vi "PhotonVision_ReadData.vi"() -> ()   [LabVIEW 2019]
uses:
  <vilib>/Rock Robotics/WPI/ThirdParty/PhotonVisionLib/TypeDef/PhotonPipelineResultType.ctl
  <vilib>/Rock Robotics/WPI/ThirdParty/PhotonVisionLib/TypeDef/PhotonTrackedTargetType.ctl
  <vilib>/Rock Robotics/WPI/ThirdParty/PhotonVisionLib/TypeDef/TargetCornerType.ctl
  <vilib>/Rock Robotics/WPI/ThirdParty/JAS_Junk/TrajLib/TypeDef/TRANSFORM3D.ctl
  <vilib>/Rock Robotics/WPI/ThirdParty/JAS_Junk/TrajLib/TypeDef/TRANSLATION3D.ctl
  <vilib>/Rock Robotics/WPI/ThirdParty/JAS_Junk/TrajLib/TypeDef/ROTATION3D.ctl
  <vilib>/Rock Robotics/WPI/ThirdParty/JAS_Junk/TrajLib/TypeDef/QUATERNION.ctl
  <vilib>/Rock Robotics/Network Tables/NT Write Boolean.vi
  <vilib>/Rock Robotics/Network Tables/NT Write Number.vi
  <vilib>/Rock Robotics/WPI/ThirdParty/PhotonVisionLib/PhotonVisionLib.lvlib
  <vilib>/Rock Robotics/WPI/ThirdParty/JAS_Junk/TrajLib/Trajectory_Library.lvlib
panel:
  out "IsConnected":bool
  out "Found Targets":bool
  in  "CameraName":string="Microsoft LifeCam HD-3000"
  out "CtrlLibDistToBestTarg\nMeters":dbl
  out "Loop Count":i32
  out "SpecificPhotonTrackedTarget":T1={"Yaw"=0.0, "Pitch"=0.0, "Area"=0.0, "Skew"=0.0, "MinAreaRectCorners"=[], "BestCameraToTarget"={"TRANSLATION3D"={"X"=0.0, "Y"=0.0, "Z"=0.0}, "ROTATION3D"={"Q_quaternion"={"R"=1.0, "V"=[0.0, 0.0, 0.0]}}, "XF"=FALSE}, "FiiducialId"=0, "AltCameraToTarget"={"TRANSLATION3D"={"X"=0.0, "Y"=0.0, "Z"=0.0}, "ROTATION3D"={"Q_quaternion"={"R"=0.0, "V"=[0.0, 0.0, 0.0]}}, "XF"=FALSE}, "PoseAmbiguity"=0.0, "DetectedCorners"=[]} {"AltCameraToTarget"."TRANSLATION3D"."Z" format="%14.3f"; "AltCameraToTarget"."TRANSLATION3D"."Y" format="%14.3f"; "AltCameraToTarget"."TRANSLATION3D"."X" format="%14.3f"; "BestCameraToTarget"."TRANSLATION3D"."Z" format="%14.3f"; "BestCameraToTarget"."TRANSLATION3D"."Y" format="%14.3f"; "BestCameraToTarget"."TRANSLATION3D"."X" format="%14.3f"}
  out "PipelineResult":T7 {"Targets"."AltCameraToTarget"."TRANSLATION3D"."Z" format="%14.3f"; "Targets"."AltCameraToTarget"."TRANSLATION3D"."Y" format="%14.3f"; "Targets"."AltCameraToTarget"."TRANSLATION3D"."X" format="%14.3f"; "Targets"."BestCameraToTarget"."TRANSLATION3D"."Z" format="%14.3f"; "Targets"."BestCameraToTarget"."TRANSLATION3D"."Y" format="%14.3f"; "Targets"."BestCameraToTarget"."TRANSLATION3D"."X" format="%14.3f"}
  out "SpecificTargetFound":bool
  out "TagTarget Index":i32
  in  "Fiiducial ID\n(April Tag Number)":i32
  out "BestTargetFound":bool
  out "BestYaw":dbl
  out "DistanceToBestTarget \nMeters":dbl
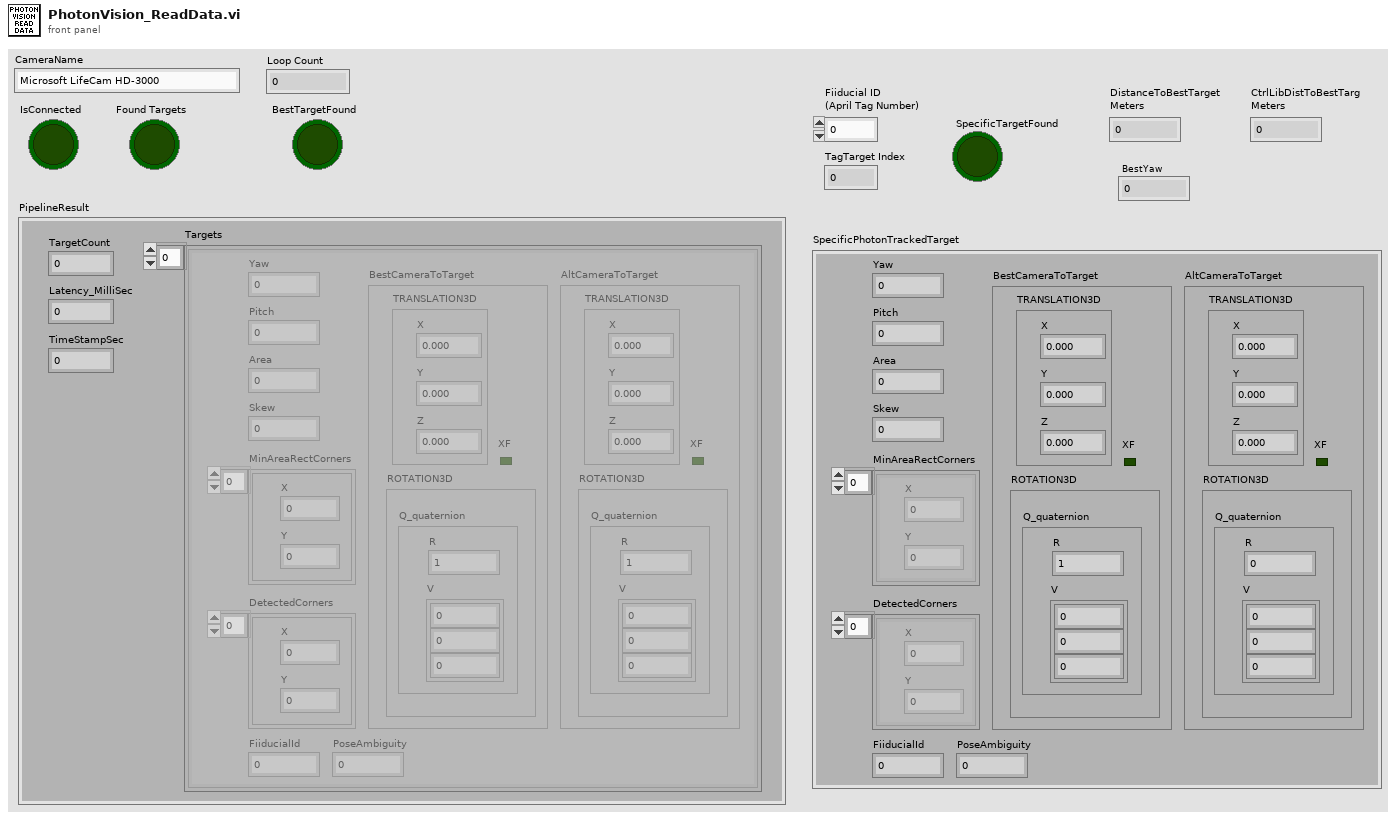
[diagram p1: front panel]
types:
  T1 = typedef "PhotonVisionLib.lvlib/PhotonTrackedTargetType.ctl" = cluster{"Yaw":dbl, "Pitch":dbl, "Area":dbl, "Skew":dbl, "MinAreaRectCorners":T2[], "BestCameraToTarget":T3, "FiiducialId":i32, "AltCameraToTarget":T3, "PoseAmbiguity":dbl, "DetectedCorners":T2[]}
  T2 = typedef "PhotonVisionLib.lvlib/TargetCornerType.ctl" = cluster{"X":dbl, "Y":dbl}
  T3 = typedef "Trajectory_Library.lvlib/TRANSFORM3D.ctl" = cluster{"TRANSLATION3D":T4, "ROTATION3D":T5, "XF":bool}
  T4 = typedef "Trajectory_Library.lvlib/TRANSLATION3D.ctl" = cluster{"X":dbl, "Y":dbl, "Z":dbl}
  T5 = typedef "Trajectory_Library.lvlib/ROTATION3D.ctl" = cluster{"Q_quaternion":T6}
  T6 = typedef "Trajectory_Library.lvlib/QUATERNION.ctl" = cluster{"R":dbl, "V":dbl[]}
  T7 = typedef "PhotonVisionLib.lvlib/PhotonPipelineResultType.ctl" = cluster{"TargetCount":i32, "Latency_MilliSec":dbl, "Targets":T1[], "TimeStampSec":dbl}
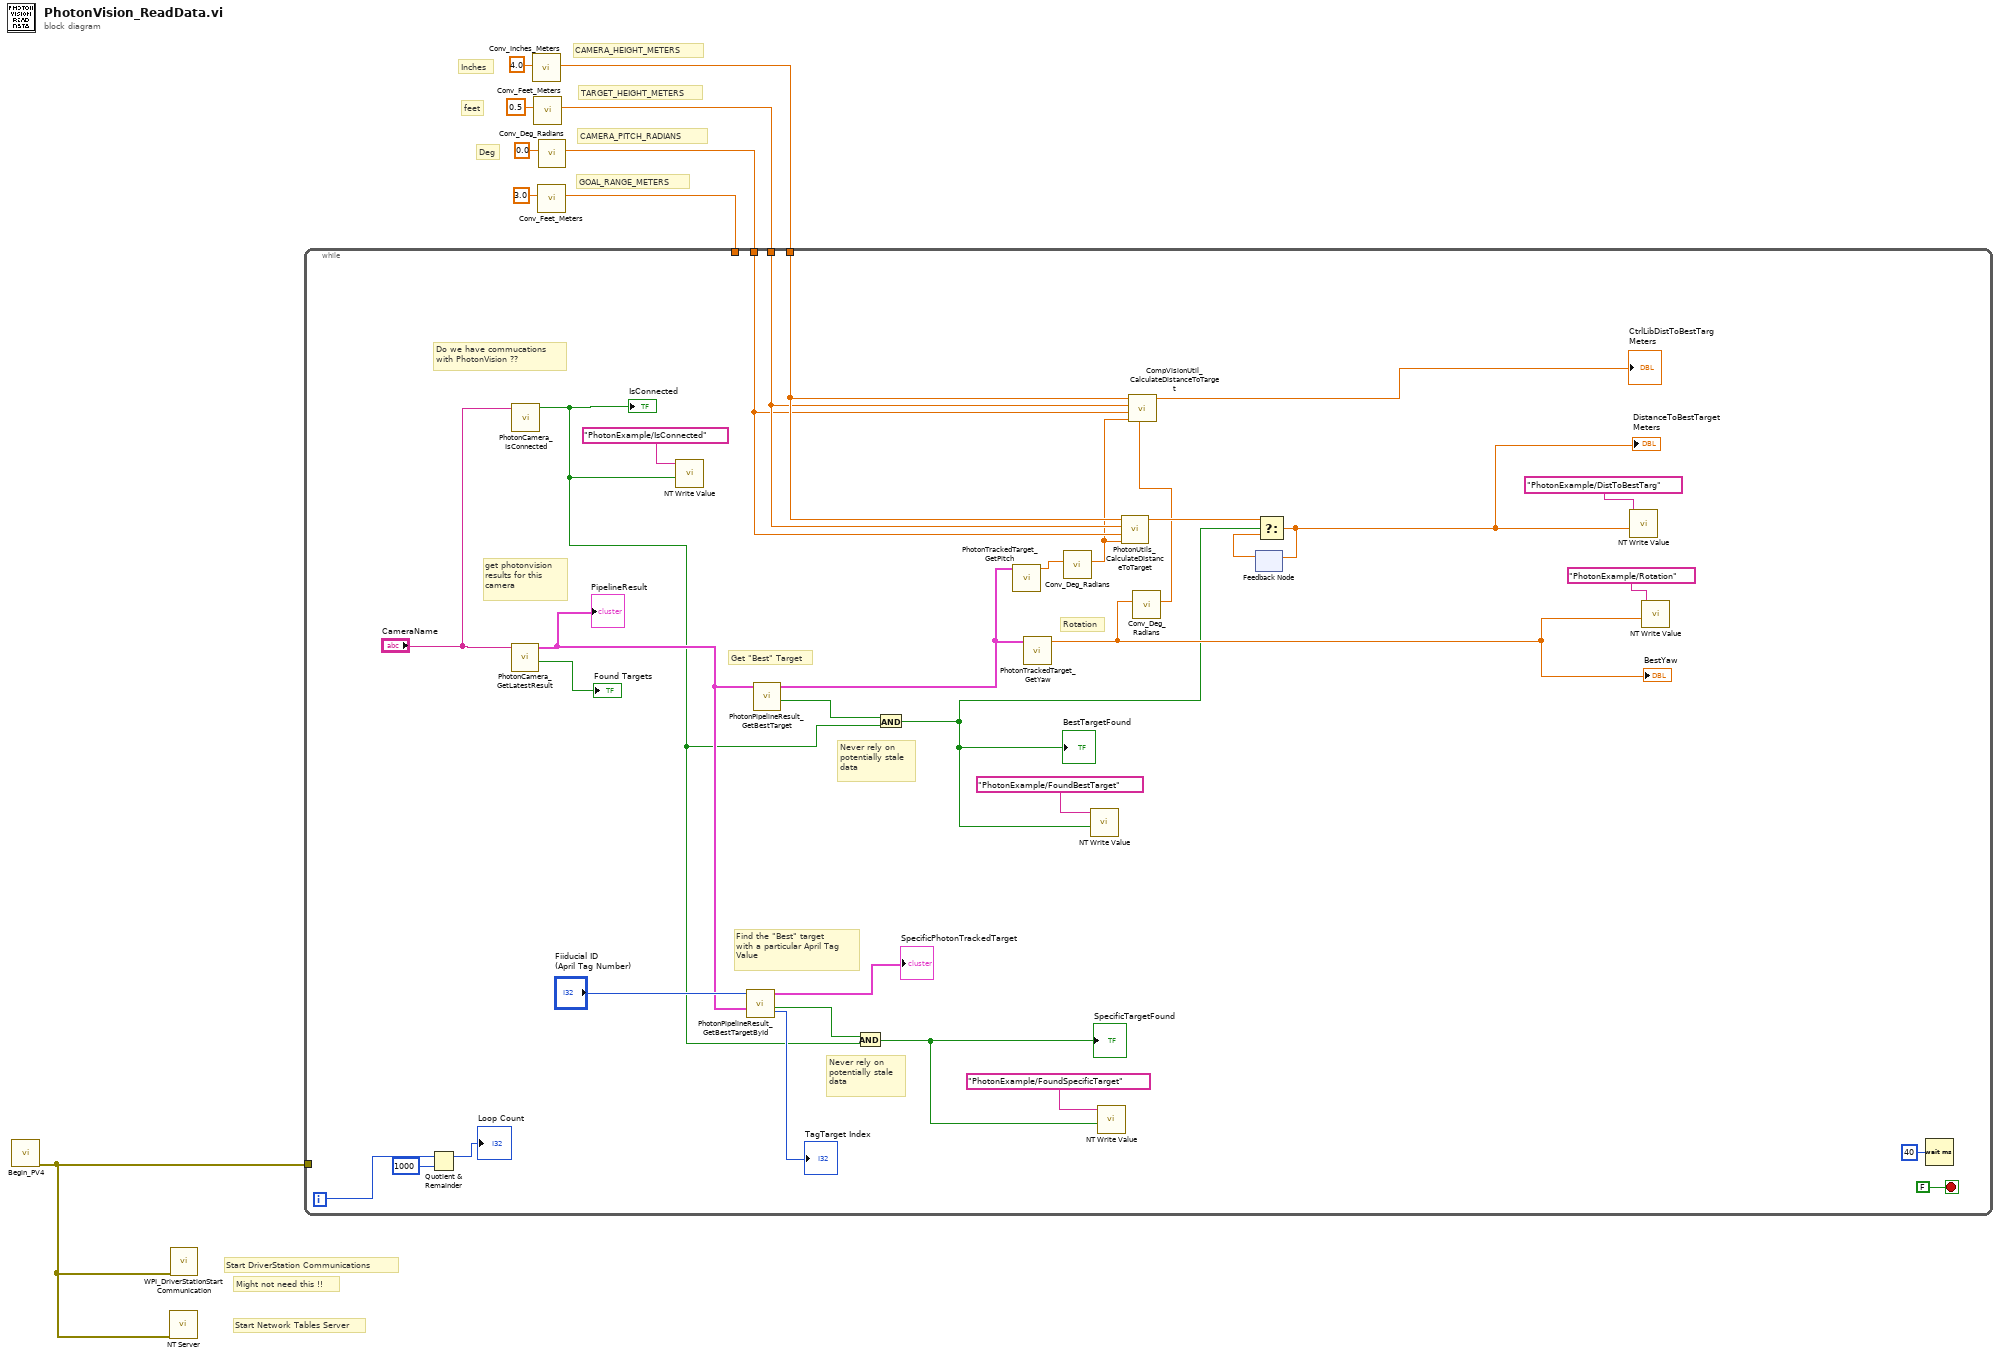
[diagram p0: block diagram]
diagram:
  # "Might not need this !!"
  # "Deg"
  # "feet"
  # "Inches"
  # "GOAL_RANGE_METERS"
  # "CAMERA_PITCH_RADIANS"
  # "TARGET_HEIGHT_METERS"
  # "CAMERA_HEIGHT_METERS"
  # "Start Network Tables Server"
  # "Start DriverStation Communications"
  n1 = call "Begin_PV4.vi"() -> ("error out"=w1:errorcluster)  [unwired: 11 in]
  n2 = call <vilib>:"NT Server.vi"("error in (no error)"=w1) -> ()  [unwired: 11 in]
  n3 = call <vilib>:"WPI_DriverStationStart Communication.vi"("error in (no error)"=w1) -> ()  [unwired: 11 in]
  n4 = call <vilib>:"Conv_Inches_Meters.vi"("INCH"=4.0) -> ("Meters"=w5:dbl)  [unwired: 10 in]
  n5 = call <vilib>:"Conv_Feet_Meters.vi"("Feet"=0.5) -> ("Meters"=w4:dbl)  [unwired: 10 in]
  n6 = call <vilib>:"Conv_Feet_Meters.vi"("Feet"=3.0) -> ("Meters"=w2:dbl)  [unwired: 10 in]
  n7 = call <vilib>:"Conv_Deg_Radians.vi"("Degress"=0.0) -> ("Radians"=w3:dbl)  [unwired: 10 in]
  n8 = while {
    tunnel: w5 -> [w24]
    tunnel: w4 -> [w23]
    tunnel: w3 -> [w22]
    tunnel: w2 -> [_]
    tunnel: w1 -> [_]
    i -> [w27]
    stop <- FALSE stop-if-true
    # "Never rely on\npotentially stale\ndata"
    # "Never rely on\npotentially stale\ndata"
    # "Do we have commucations\nwith PhotonVision ??"
    # "Find the \"Best\" target\nwith a particular April Tag\nValue"
    # "Get \"Best\" Target"
    # "Rotation"
    # "get photonvision\nresults for this\ncamera"
    n9 = Quotient & Remainder(x=w27, y=1000) -> (x-y*floor(x/y)=→"Loop Count":i32)  [unwired: 1 out]
    n10 = call <vilib>:"PhotonCamera_GetLatestResult.vi"("CameraName"="CameraName") -> ("HasTargets"=→"Found Targets":bool, "PipelineResult"=w31:T7)  [unwired: 9 in]
    "PipelineResult" <- w31
    n11 = call <vilib>:"PhotonCamera_IsConnected.vi"("CameraName"="CameraName") -> ("IsConnected"=w10:bool)  [unwired: 10 in]
    "IsConnected" <- w10
    n12 = call-poly <vilib>:"NT Write Value.vi"("Boolean"=w10, "Name"="PhotonExample/IsConnected") -> ()  [unwired: 9 in, 1 out]
    n13 = call <vilib>:"PhotonPipelineResult_GetBestTargetById.vi"("PhotonPipelineResult"=w31, "FiducialId"="Fiiducial ID\n(April Tag Number)") -> ("Target Found"=w11:bool, "PhotonTrackedTarget"=→"SpecificPhotonTrackedTarget":T1, "Target Index"=→"TagTarget Index":i32)  [unwired: 7 in]
    n14 = call <vilib>:"PhotonPipelineResult_GetBestTarget.vi"("PhotonPipelineResult"=w31) -> ("TargetFound"=w14:bool, "PhotonTrackedTarget"=w32:T1)  [unwired: 9 in]
    n15 = And(x=w11, y=w10) -> (x .and. y?=w12:bool)
    "SpecificTargetFound" <- w12
    n16 = And(x=w14, y=w10) -> (x .and. y?=w13:bool)
    "BestTargetFound" <- w13
    n17 = call <vilib>:"PhotonTrackedTarget_GetPitch.vi"("TrackedTarget"=w32) -> ("Pitch"=w34:dbl)  [unwired: 10 in]
    n18 = call <vilib>:"PhotonTrackedTarget_GetYaw.vi"("TrackedTarget"=w32) -> ("Yaw"=w20:dbl)  [unwired: 10 in]
    "BestYaw" <- w20
    n19 = call <vilib>:"Conv_Deg_Radians.vi"("Degress"=w34) -> ("Radians"=w21:dbl)  [unwired: 10 in]
    n20 = call-poly <vilib>:"NT Write Value.vi"("Boolean"=w13, "Name"="PhotonExample/FoundBestTarget") -> ()  [unwired: 9 in, 1 out]
    n21 = call-poly <vilib>:"NT Write Value.vi"("Boolean"=w12, "Name"="PhotonExample/FoundSpecificTarget") -> ()  [unwired: 9 in, 1 out]
    n22 = call <vilib>:"PhotonUtils_CalculateDistanceToTarget.vi"("TargetPitch_Radians"=w21, "CameraPitch_Radians"=w22, "TargetHeight_Meters"=w23, "CameraHeight_Meters"=w24) -> ("DistanceToTarget_Meters"=w37:dbl)  [unwired: 7 in]
    n23 = call <vilib>:"Conv_Deg_Radians.vi"("Degress"=w20) -> ("Radians"=w19:dbl)  [unwired: 10 in]
    n24 = call <vilib>:"CompVisionUtil_CalculateDistanceToTarget.vi"("TargetYawRadians"=w19, "targetPitch_Radians"=w21, "cameraPitch_Radians"=w22, "targetHeight_Meters"=w23, "cameraHeight_Meters"=w24) -> ("DistanceToTarget_Meters"=→"CtrlLibDistToBestTarg\nMeters":dbl)  [unwired: 6 in]
    n25 = feedback #1() -> (w35:dbl)  [unwired: 1 in]
    n26 = Select(t=w37, s=w13, f=w35) -> (s? t:f=w36:dbl)
    "DistanceToBestTarget \nMeters" <- w36
    n27 = feedback-in #1(w36) -> ()
    n28 = call-poly <vilib>:"NT Write Value.vi"("Numeric"=w36, "Name"="PhotonExample/DistToBestTarg") -> ()  [unwired: 9 in, 1 out]
    n29 = call-poly <vilib>:"NT Write Value.vi"("Numeric"=w20, "Name"="PhotonExample/Rotation") -> ()  [unwired: 9 in, 1 out]
    n30 = Wait (ms)(milliseconds to wait=u32 40) -> ()  [unwired: 1 out]
  }
